vi "Is stdin queue valid.vi"(1 "stdin packet queue":refnum<queue>) -> (0 "valid?":bool)   [LabVIEW 2020, in "NI_SFTP.lvlib" / "Low Level Connection.lvclass"]
uses:
  <vilib>/net/SFTP/Low Level Connection/Low Level Connection.lvclass
  <vilib>/Array/Bytestream/Bytestream.lvclass
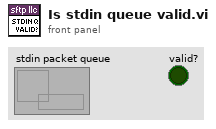
[diagram p1: front panel]
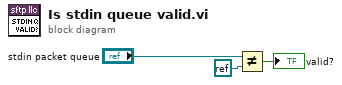
[diagram p0: block diagram]
diagram:
  n1 = Not Equal?(x="stdin packet queue", y=refnum<k0> refnum) -> (x != y?=→"valid?":bool)
